vi "Delete Targets.vi"(8 "error in (no error)":errorcluster, 10 "Targets":string[](array[string]), 11 "State in":refnum<class "State.lvclass">) -> (0 "error out":errorcluster, 3 "State out":refnum<class "State.lvclass">)   [LabVIEW 2015, in "State.lvclass"]
uses:
  State.lvclass
  State.lvclass/State.ctl
  Termination/Termination.lvclass/Termination.ctl
  Termination/Read Link to.vi
  Termination/Termination.lvclass
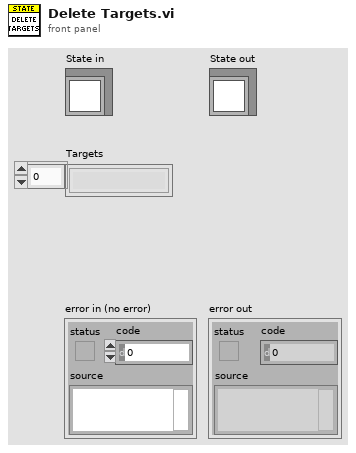
[diagram p1: front panel]
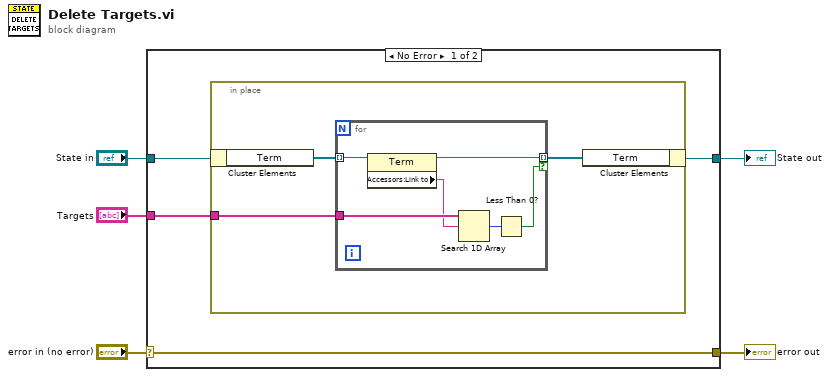
[diagram p0: block diagram]
diagram:
  n1 = case shown="No Error" "error in (no error)" {
    selector: "error in (no error)" -> [w9 w20]
    tunnel: [w9 w20] -> w4
    tunnel: [w7 w19] -> w2
    tunnel: "State in" -> [w8 w19]
    tunnel: "Targets" -> [w6 _]
    frame No Error {
      n2 = in-place {
        in-place-border: w6 -> [w11]
        n3 = in-place-cluster #1(w8) -> ("Term"=w12:refnum<class "Termination.lvclass">[])
        n4 = for {
          tunnel: w12 -> [w18] mode=indexing
          tunnel: w11 -> [w17]
          tunnel: [w15] -> w10 mode=indexing if=w13
          n5 = property class="Term"(reference=w18) -> (reference out=w15:refnum<class "Termination.lvclass">, "Accessors:Link to"=w16:string)  [unwired: 1 in, 1 out]
          n6 = Search 1D Array(1D array=w17, element=w16) -> (index of element=w14:i32)  [unwired: 1 in]
          n7 = Less Than 0?(x=w14) -> (x < 0?=w13:bool)
        }
        n8 = in-place-cluster #1("Term"=w10) -> (w7:refnum<class "State.lvclass">)
      }
    }
    frame Error {
    }
  }
  "error out" <- w4
  "State out" <- w2
